vi "VI Launcher - no GUI.vi"   [LabVIEW 2011]
doc: "This VI will launch a daemon who's front panel is not loaded into memory. The shipping version of this VI does not work. You must modify it to apprpriately manage the VI reference to the daemon. \n\nAAL 9/09"
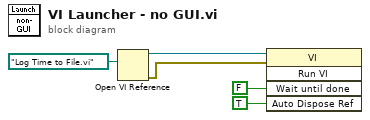
[diagram p0: block diagram]
diagram:
  n1 = Open VI Reference(vi path=path "Log Time to File.vi") -> (vi reference=w2:refnum<vi>, error out=w1:errorcluster)  [unwired: 1 in, 4 out]
  n2 = invoke class="VI" method="Run VI"(reference=w2, error in=w1, "Wait until done"=FALSE ("Wait Until Done"), "Auto Dispose Ref"=TRUE ("Auto Dispose Reference")) -> ()  [unwired: 1 in, 5 out]
